vi "PathPlanner_PathFinder_ExtractPathSub1.vi"(9 "SStart":T1, 10 "SGoal":T1, 11 "PathPoints In":T1[](array[typedef])) -> (3 "Path Points Out":T1[](array[typedef]))   [LabVIEW 2019]
uses:
  PathPlannerLib24/TypeDef/PathPlannerFinderGridPosition.ctl
  PathPlannerLib24/VI/PathPlanner_GridPosition_Get.vi
  PathPlannerLib24/VI/PathPlanner_GridPosition_New.vi
  PathPlannerLib24/VI/PathPlanner_PathFinder_Globals.vi
  PathPlannerLib24/PathPlanner24.lvlib
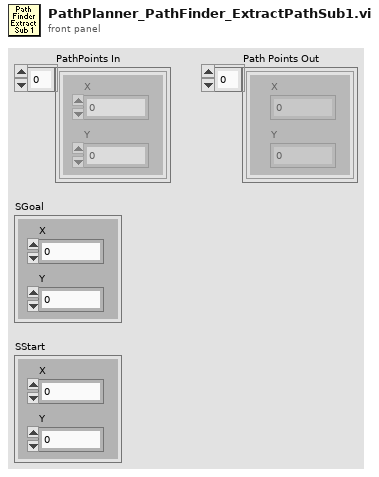
[diagram p1: front panel]
types:
  T1 = typedef "PathPlanner24.lvlib/PathPlannerFinderGridPosition.ctl" = cluster{"X":i32, "Y":i32}
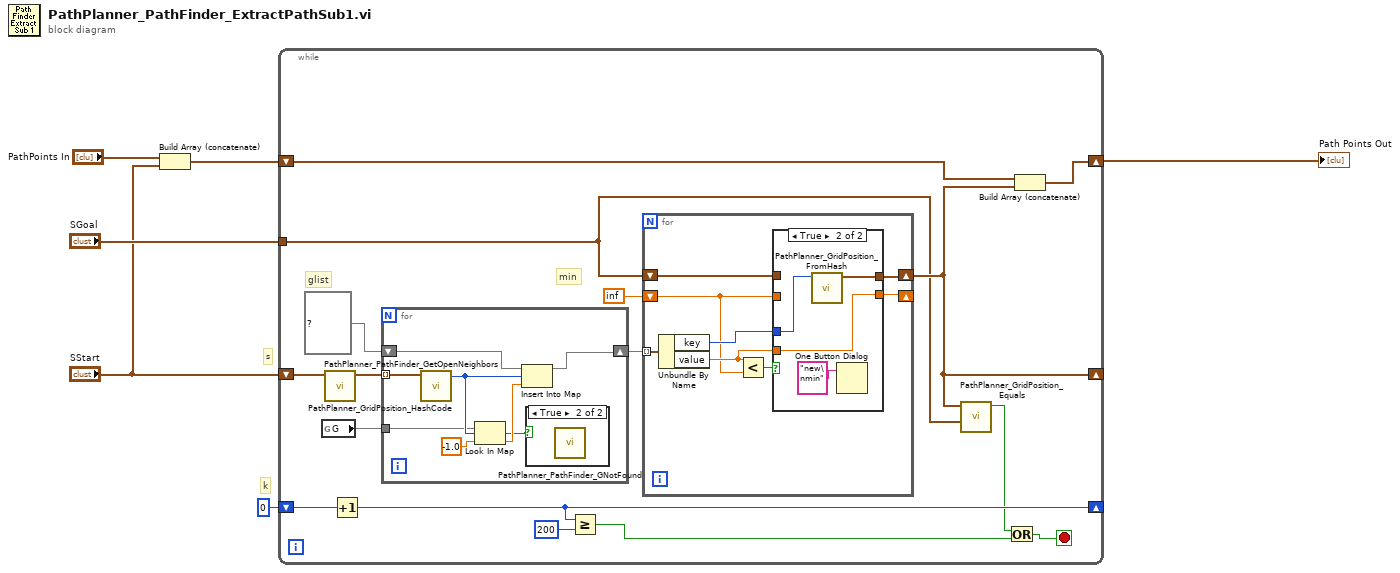
[diagram p0: block diagram]
diagram:
  # "s"
  # "k"
  n1 = Build Array (concatenate)("PathPoints In", "SStart") -> (w1:T1[])
  n2 = while {
    shift-right: [w21] -> _
    shift-left: 0 -> [w22]
    tunnel: "SGoal" -> [w9]
    shift-right: [w10] -> _
    shift-left: "SStart" -> [w19]
    shift-right: [w13] -> w6
    shift-left: w1 -> [w14]
    stop <- w12 stop-if-true
    # "min"
    # "glist"
    n3 = global read "PathPlanner_PathFinder_Globals.vi" "G"() -> (w7:map{i32, dbl})
    n4 = call "PathPlanner_PathFinder_GetOpenNeighbors.vi"("GridPosition S"=w19) -> ("Open Neighbors"=w18:T1[])  [unwired: 10 in]
    n5 = Increment(x=w22) -> (x+1=w21:i32)
    n6 = for {
      tunnel: w18 -> [w44] mode=indexing
      shift-right: [w39] -> w16
      shift-left: map{i32, dbl} {} ("G") -> [w42]
      tunnel: w7 -> [w38]
      n7 = call "PathPlanner_GridPosition_HashCode.vi"("GridPosition"=w44) -> ("HashCode"=w41:i32)  [unwired: 10 in]
      n8 = Look In Map(map=w38, key=w41, default value=-1.0) -> (key not found?=w37:bool, value=w40:dbl)
      n9 = Insert Into Map(map in=w42, key=w41, value=w40) -> (map out=w39:map{i32, dbl})  [unwired: 2 out]
      n10 = case shown="True" w37 {
        frame False {
        }
        frame True {
          n11 = call "PathPlanner_PathFinder_GNotFound.vi"() -> ()  [unwired: 12 in]
        }
      }
    }
    n12 = Greater Or Equal?(x=w21, y=200) -> (x >= y?=w11:bool)
    n13 = for {
      tunnel: w16 -> [w30] mode=indexing
      shift-right: [w27] -> w10
      shift-left: w9 -> [w24]
      shift-right: [w26] -> _
      shift-left: inf -> [w23]
      n14 = Unbundle By Name(w30) -> ("key"=w28:i32, "value"=w25:dbl)
      n15 = Less?(x=w25, y=w23) -> (x < y?=w29:bool)
      n16 = case shown="True" w29 {
        tunnel: w28 -> [_ w36]
        tunnel: [w32 w35] -> w27
        tunnel: [w31 w34] -> w26
        tunnel: w25 -> [_ w34]
        tunnel: w24 -> [w32 _]
        tunnel: w23 -> [w31 _]
        frame False {
        }
        frame True {
          n17 = call "PathPlanner_GridPosition_FromHash.vi"("Hash"=w36) -> ("GridPosition"=w35:T1)  [unwired: 10 in]
          n18 = One Button Dialog(message="new\nmin") -> ()  [unwired: 1 in, 1 out]
        }
      }
    }
    n19 = call "PathPlanner_GridPosition_Equals.vi"("Other GridPosition"=w9, "GridPosition"=w10) -> ("Equal"=w8:bool)  [unwired: 9 in]
    n20 = Or(x=w8, y=w11) -> (x .or. y?=w12:bool)
    n21 = Build Array (concatenate)(w14, w10) -> (w13:T1[])
  }
  "Path Points Out" <- w6
